vi "Read RP Configuration.vi"(8 "error in (no error)":errorcluster, 11 "Red Pitaya Digitizer in":refnum<class "Red Pitaya Digitizer.lvclass">) -> (0 "error out":errorcluster, 2 "Configuration":T1={"Ranges"=[20.0, 20.0], "Output frequency 1"=50000.0, "Output frequency 2"=50000.0, "Pre-trigger samples"=-100000, "Post-trigger samples"=11534336, "Desimation rate"=125, "Delayed start"=571428} {"Delayed start" format="0x%x (%d)"; "Post-trigger samples" format="0x%x (%d)"; "Pre-trigger samples" format="0x%x (%d)"; "Output frequency 2" format="%#_6p"; "Output frequency 1" format="%#_6p"; "Ranges" format="%#_12p"}, 3 "Red Pitaya Digitizer out":refnum<class "Red Pitaya Digitizer.lvclass">)   [LabVIEW 2015, in "Red Pitaya Digitizer.lvclass"]
uses:
  Red Pitaya Digitizer.lvclass
  RP Configuration.ctl
  Measure_core/Measure Object/Measure Object.lvclass/Measure Object.ctl
  Measure_core/Measure Object/Read Configuration.vi
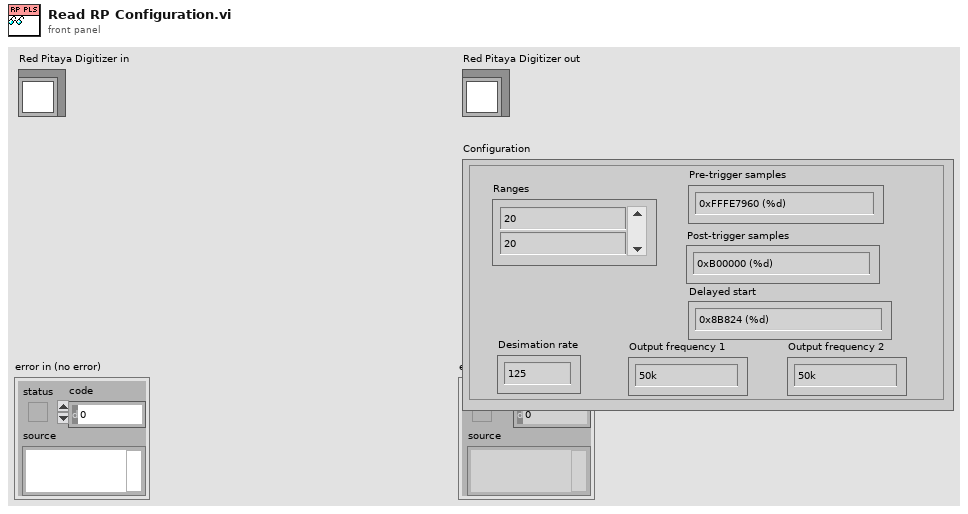
[diagram p1: front panel]
types:
  T1 = typedef "RP Configuration.ctl" = cluster{"Ranges":dbl[], "Output frequency 1":dbl, "Output frequency 2":dbl, "Pre-trigger samples":i32, "Post-trigger samples":u64, "Desimation rate":u64, "Delayed start":u64}
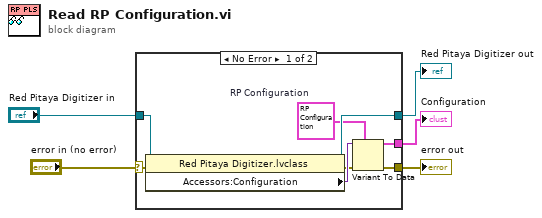
[diagram p0: block diagram]
diagram:
  n1 = case shown="No Error" "error in (no error)" {
    selector: "error in (no error)" -> [w10 w14]
    tunnel: [w7 w14] -> w4
    tunnel: [w12 w15] -> w2
    tunnel: "Red Pitaya Digitizer in" -> [w13 w15]
    tunnel: [w8 _] -> w1
    frame No Error {
      w9 = T1 {"Ranges"=[20.0, 20.0], "Output frequency 1"=50000.0, "Output frequency 2"=50000.0, "Pre-trigger samples"=-100000, "Post-trigger samples"=11534336, "Desimation rate"=125, "Delayed start"=571428}  # RP Configuration
      n2 = property class="Red Pitaya Digitizer.lvclass"(reference=w13, error in=w10) -> (reference out=w12:refnum<class "Red Pitaya Digitizer.lvclass">, error out=w6:errorcluster, "Accessors:Configuration"=w11:variant)
      n3 = Variant To Data(error in=w6, type=w9, Variant=w11) -> (data=w8:T1, error out=w7:errorcluster)
    }
    frame Error {
    }
  }
  "error out" <- w4
  "Red Pitaya Digitizer out" <- w2
  "Configuration" <- w1
